vi "Linear Interpolation VtoGPM.vi"(5 "V to GPM":dbl[][](array[numeric])=[[0.483, 1.17], [0.806, 1.93], [1369.0, 3.3], [2.015, 4.87], [2.576, 6.12], [2.897, 6.95], [3.048, 7.31], [3.296, 7.7]] format="%0.3f", 10 "V":dbl) -> (2 "GPM":dbl)   [LabVIEW 2009]
uses:
  <vilib>/gmath/NI_Gmath.lvlib
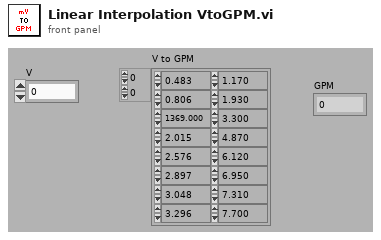
[diagram p1: front panel]
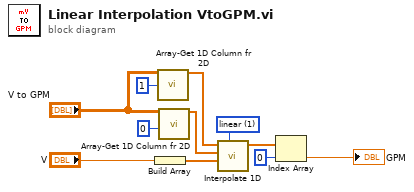
[diagram p0: block diagram]
diagram:
  w11 = 1 items=["nearest", "linear", "spline", "cubic Hermite", "Lagrange"] ("method")
  n1 = Build Array("V") -> (w8:dbl[])
  n2 = call "Array-Get 1D Column fr 2D.vi"("2D Array Data"="V to GPM", "column index"=1) -> ("Column Data"=w2:dbl[])  [unwired: 13 in]
  n3 = call "Array-Get 1D Column fr 2D.vi"("2D Array Data"="V to GPM", "column index"=0) -> ("Column Data"=w3:dbl[])  [unwired: 13 in]
  n4 = call <vilib>:"Interpolate 1D.vi"("method"=w11, "xi"=w8, "X"=w3, "Y"=w2) -> ("yi"=w7:dbl[])  [unwired: 5 in, 2 out]
  n5 = Index Array(array=w7, index=0) -> (element=→"GPM":dbl)
